vi "action.vi"(0 "HGF_FGV_VisitSelection":refnum<class "HGF_FGV_VisitSelection.lvclass">, 2 "Objects":refnum<class>[](array[class]), 5 "error in (no error)":errorcluster) -> (14 "dup HGF_FGV_VisitSelection":refnum<class "HGF_FGV_VisitSelection.lvclass">, 16 "dup Objects":refnum<class>[](array[class]), 19 "error out":errorcluster)   [LabVIEW 2012, in "HGF_FGV.lvlib" / "HGF_FGV_VisitSelection.lvclass"]
doc: "Apply Visitors action to selected objects in FGV instance."
uses:
  HGF_FGV_VisitSelection.lvclass
  HGF_Visitable/HGF_Visitable.lvclass
  HGF_FGV_VisitSelection.lvclass/HGF_FGV_VisitSelection.ctl
  HGF_FGV_Visitor/HGF_FGV_Visitor.lvclass
  HGF_Visitor/HGF_Visitor.lvclass
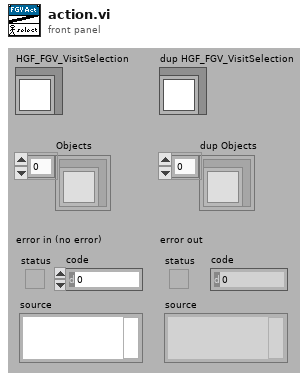
[diagram p1: front panel]
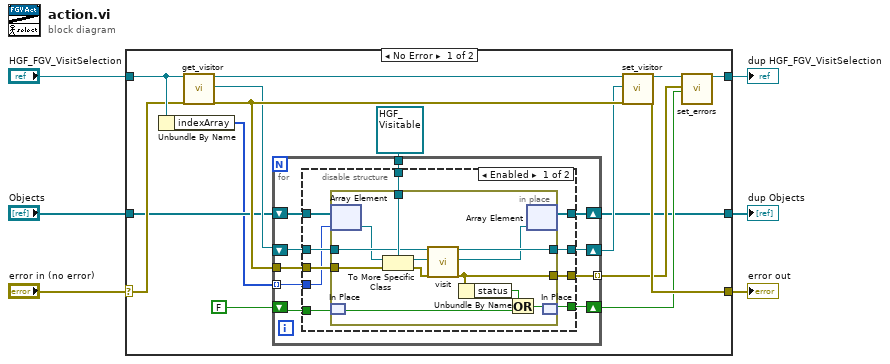
[diagram p0: block diagram]
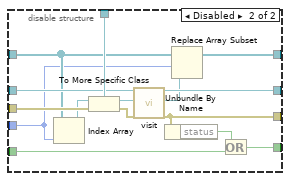
[diagram p2: hidden frame]
diagram:
  n1 = case shown="No Error" "error in (no error)" {
    selector: "error in (no error)" -> [w20 w72]
    tunnel: [w19 w72] -> w5
    tunnel: [w12 w71] -> w3
    tunnel: "HGF_FGV_VisitSelection" -> [w22 w71]
    tunnel: [w7 w70] -> w2
    tunnel: "Objects" -> [w9 w70]
    frame No Error {
      n2 = Unbundle By Name(w22) -> ("indexArray"=w8:u32[])
      n3 = call "get_visitor.vi"("HGF_FGV_Visitor"=w22, "error in (no error)"=w20) -> ("dup HGF_FGV_Visitor"=w21:refnum<class "HGF_FGV_VisitSelection.lvclass">, "visitor"=w16:refnum<class "HGF_Visitor.lvclass">, "error out"=w17:errorcluster)  [unwired: 15 out]
      n4 = for {
        tunnel: refnum<class "HGF_Visitable.lvclass"> refnum ("HGF_Visitable.lvclass") -> [w32]
        shift-right: [w29] -> w15
        shift-left: w16 -> [w30]
        tunnel: w17 -> [w31]
        tunnel: [w28] -> w11 mode=indexing
        shift-right: [w27] -> w10
        shift-left: FALSE -> [w26]
        tunnel: w8 -> [w23] mode=indexing
        shift-right: [w24] -> w7
        shift-left: w9 -> [w25]
        n5 = disable-structure shown="Enabled" {
          disable-tunnel: w32 -> [w42 w67]
          disable-tunnel: w31 -> [w41 w66]
          disable-tunnel: w30 -> [w40 w65]
          disable-tunnel: [w39 w64] -> w29
          disable-tunnel: [w38 w63] -> w28
          disable-tunnel: [w33 w62] -> w27
          disable-tunnel: w26 -> [w34 w60]
          disable-tunnel: w25 -> [w36 w58]
          disable-tunnel: [w35 w57] -> w24
          disable-tunnel: w23 -> [w37 w55]
          frame Enabled {
            n6 = in-place {
              in-place-border: w42 -> [w52]
              in-place-border: w41 -> [w51]
              in-place-border: w40 -> [w50]
              in-place-border: [w49] -> w39
              in-place-border: [w48] -> w38
              n7 = in-place-array #1(w36, w37) -> (w46:refnum<class>)
              n8 = in-place-match #2(w34) -> (w43:bool)
              n9 = To More Specific Class(target class=w52, reference=w46, error in=w51) -> (specific class reference=w53:refnum<class "HGF_Visitable.lvclass">, error out=w54:errorcluster)
              n10 = call "visit.vi"("HGF_Visitor"=w50, "HGF_Visitable"=w53, "error in (no error)"=w54) -> ("dup HGF_Visitor"=w49:refnum<class "HGF_Visitor.lvclass">, "dup HGF_Visitable"=w45:refnum<class "HGF_Visitable.lvclass">, "error out"=w48:errorcluster)  [unwired: 14 out]
              n11 = Unbundle By Name(w48) -> ("status"=w47:bool)
              n12 = Or(x=w47, y=w43) -> (x .or. y?=w44:bool)
              n13 = in-place-array #1(w45) -> (w35:refnum<class>[])  [unwired: 1 out]
              n14 = in-place-match #2(w44) -> (w33:bool)
            }
          }
          frame Disabled {
            n15 = Index Array(array=w58, index=w55) -> (element=w59:refnum<class>)
            n16 = To More Specific Class(target class=w67, reference=w59, error in=w66) -> (specific class reference=w68:refnum<class "HGF_Visitable.lvclass">, error out=w69:errorcluster)
            n17 = call "visit.vi"("HGF_Visitor"=w65, "HGF_Visitable"=w68, "error in (no error)"=w69) -> ("dup HGF_Visitor"=w64:refnum<class "HGF_Visitor.lvclass">, "dup HGF_Visitable"=w56:refnum<class "HGF_Visitable.lvclass">, "error out"=w63:errorcluster)  [unwired: 14 in]
            n18 = Unbundle By Name(w63) -> ("status"=w61:bool)
            n19 = Replace Array Subset(array=w58, new element=w56, index=w55) -> (w57:refnum<class>[])
            n20 = Or(x=w61, y=w60) -> (x .or. y?=w62:bool)
          }
        }
      }
      n21 = call "set_visitor.vi"("HGF_FGV_Visitor"=w21, "visitor"=w15, "error in (no error)"=w17) -> ("dup HGF_FGV_Visitor"=w13:refnum<class "HGF_FGV_VisitSelection.lvclass">, "error out"=w19:errorcluster)  [unwired: 15 out]
      n22 = call "set_errors.vi"("HGF_FGV_Visitor"=w13, "Errors"=w11, "error"=w10) -> ("dup HGF_FGV_Visitor"=w12:refnum<class "HGF_FGV_VisitSelection.lvclass">)  [unwired: 1 in, 15 out]
    }
    frame Error {
    }
  }
  "error out" <- w5
  "dup HGF_FGV_VisitSelection" <- w3
  "dup Objects" <- w2
